vi "WriteHeaderFile.vi"(8 "error in (no error)":errorcluster, 10 "HeadersFileName":path, 11 "ScanPar":T1={"Entête"="", "Scan list"=[], "NbCourbe"=1, "IndCourbe"=0, "NomDon"=["RTêta;", "X&Y;"], "Session "=0, "Date"="", "Time"="", "VarParams"=[], "UserName"="", "ScanTableSize"=[], "VarPar list"=[], "DescKeyword"=""} caption="ScanParams") -> (0 "error out":errorcluster)   [LabVIEW 2019]
doc: "Ce VI sauvegarde les données d'acquisition pour en garder une copie de sécurité qui peut être rappeller en cas de panne."
uses:
  Interface Class/ScanParams.ctl
  Interface Class/Interface.lvclass
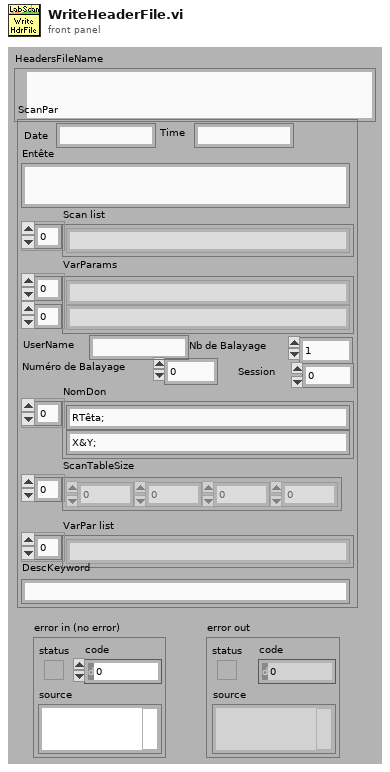
[diagram p1: front panel]
types:
  T1 = typedef "Interface.lvclass/ScanParams.ctl" = cluster{"Entête":string, "Scan list":string[], "NbCourbe":i32, "IndCourbe":i64, "NomDon":string[], "Session ":i32, "Date":string, "Time":string, "VarParams":string[][], "UserName":string, "ScanTableSize":i32[], "VarPar list":string[], "DescKeyword":string}
  T2 = enum16{"open", "replace", "create", "open or create", "replace or create", "replace or create with confirmation"}
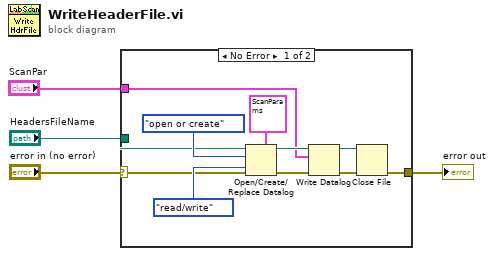
[diagram p0: block diagram]
diagram:
  n1 = case shown="No Error" "error in (no error)" {
    selector: "error in (no error)" -> [w7 w16]
    tunnel: [w5 w16] -> w3
    tunnel: "ScanPar" -> [w8 _]
    tunnel: "HeadersFileName" -> [w6 _]
    frame No Error {
      n2 = Open/Create/Replace Datalog(5:T1 {"Entête"="", "Scan list"=[], "NbCourbe"=0, "IndCourbe"=0, "NomDon"=[], "Session "=0, "Date"="", "Time"="", "VarParams"=[], "UserName"="", "ScanTableSize"=[], "VarPar list"=[], "DescKeyword"=""} ("HdrSaf"), 8:w7, 9:enum16{"read/write", "read-only", "write-only"}."read/write" ("accès (0 : read/write)"), 10:T2."open or create" ("opération (0 : open)"), 11:w6) -> (0:w14:errorcluster, 3:w15:refnum<k1>)  [unwired: 1 in, 1 out]
      n3 = Write Datalog(4:w14, 6:w8, 7:w15) -> (0:w12:errorcluster, 3:w13:refnum<k1>)
      n4 = Close File(refnum=w13, error in=w12) -> (error out=w5:errorcluster)  [unwired: 1 out]
    }
    frame Error {
    }
  }
  "error out" <- w3
